vi "setSerializedData.vi"(0 "reference":refnum<class "UseCaseNode.lvclass">, 1 "parent":refnum<class "AbstractNode.lvclass">, 2 "children":refnum<class "AbstractNode.lvclass">[](array[class]), 3 "xmlOut":string, 5 "error in (no error)":errorcluster) -> (14 "reference out":refnum<class "UseCaseNode.lvclass">, 19 "error out":errorcluster)   [LabVIEW 2014, in "UseCaseNode.lvclass"]
doc: "setSerializedData"
uses:
  <resource>/Framework/Providers/Open_GDS/UML/UseCaseNode_class/UseCaseNode.lvclass
  <resource>/Framework/Providers/Open_GDS/UML/AbstractNode_class/AbstractNode.lvclass
  <resource>/Framework/Providers/Open_GDS/UML/General/Rectangle/Rectangle Rectangle2D.ctl
  <resource>/Framework/Providers/Open_GDS/UML/MultiLineString_class/MultiLineString.lvclass
  <resource>/Framework/Providers/Open_GDS/UML/RectangularNode_class/RectangularNode.lvclass
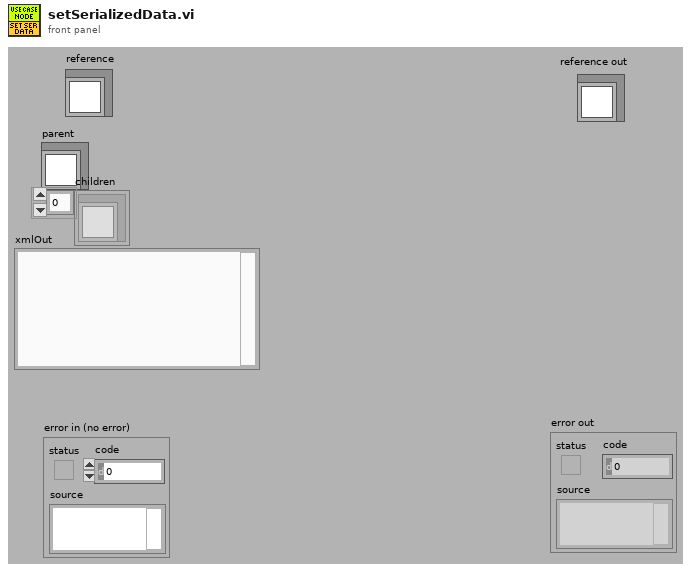
[diagram p1: front panel]
types:
  T1 = typedef "Rectangle Rectangle2D.ctl" = cluster{"x":dbl, "y":dbl, "width":dbl, "height":dbl}
  T2 = cluster{"Base class":cluster{"Base class":cluster{"parent":refnum<k1>, "children":refnum<k1>[]}, "bounds":T1}, "name":refnum<k1>, "DEFAULT_WIDTH":i32, "DEFAULT_HEIGHT":i32}
  T3 = cluster{"Attributes":cluster{"Base class":cluster{"Base class":cluster{"parent":refnum<k1>, "children":refnum<k1>[]}, "bounds":T1}, "name":refnum<k1>, "DEFAULT_WIDTH":i32, "DEFAULT_HEIGHT":i32}, string}
  T4 = typedef "UseCaseNode.lvclass/ObjectAttributes.ctl" = cluster{"name":refnum<class "MultiLineString.lvclass">, "DEFAULT_WIDTH":i32, "DEFAULT_HEIGHT":i32}
  T5 = typedef "RectangularNode.lvclass/ObjectAttributes.ctl" = cluster{"bounds":T1}
  T6 = typedef "AbstractNode.lvclass/ObjectAttributes.ctl" = cluster{"parent":refnum<class "AbstractNode.lvclass">, "children":refnum<class "AbstractNode.lvclass">[], "Hidden":bool}
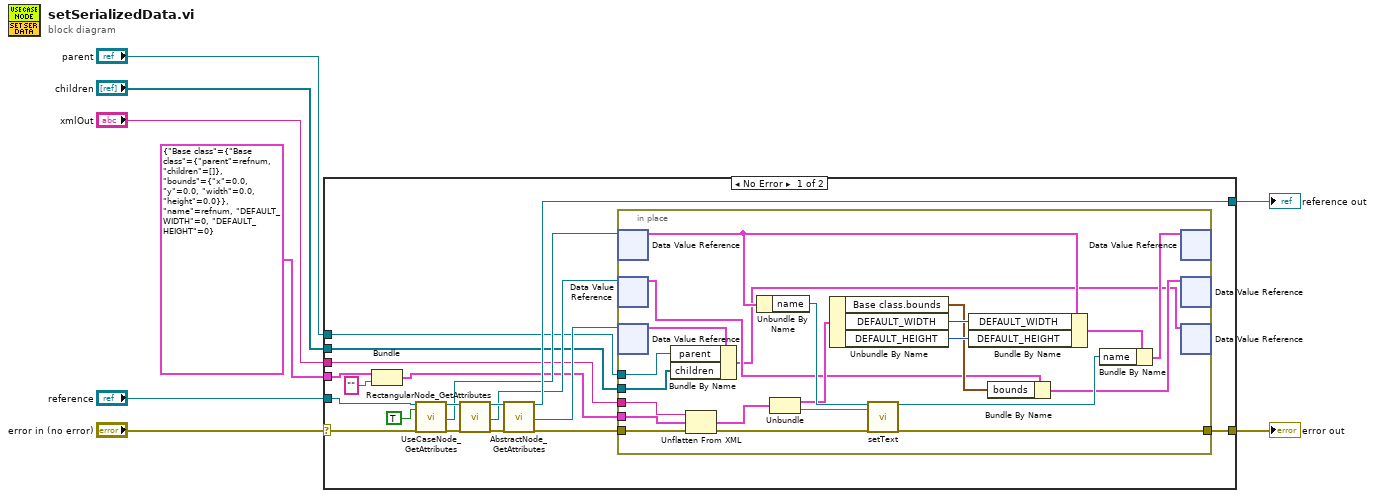
[diagram p0: block diagram]
diagram:
  n1 = case shown="No Error" "error in (no error)" {
    selector: "error in (no error)" -> [w26 w50]
    tunnel: "reference" -> [w27 w51]
    tunnel: [w25 w50] -> w6
    tunnel: [w24 w51] -> w5
    tunnel: "xmlOut" -> [w11 _]
    tunnel: "parent" -> [w10 _]
    tunnel: "children" -> [w9 _]
    tunnel: T2 {"Base class"={"Base class"={"parent"=refnum, "children"=[]}, "bounds"={"x"=0.0, "y"=0.0, "width"=0.0, "height"=0.0}}, "name"=refnum, "DEFAULT_WIDTH"=0, "DEFAULT_HEIGHT"=0} ("Attributes") -> [w22 _]
    frame No Error {
      n2 = Bundle("Attributes"=w22, "") -> (w12:T3)  [unwired: 1 out]
      n3 = call <resource>:"UseCaseNode_GetAttributes.vi"("reference in"=w27, "OnlyGetDvrReference(False)"=TRUE, "error in (no error)"=w26) -> ("reference out"=w20:refnum<class "UseCaseNode.lvclass">, "DataRef"=w16:refnum<data-value>, "error out"=w19:errorcluster)  [unwired: 13 in, 1 out]
      n4 = call <resource>:"RectangularNode_GetAttributes.vi"("reference in"=w20, "error in (no error)"=w19) -> ("reference out"=w18:refnum<class "UseCaseNode.lvclass">, "DataRef"=w15:refnum<data-value>, "error out"=w17:errorcluster)  [unwired: 14 in, 1 out]
      n5 = call <resource>:"AbstractNode_GetAttributes.vi"("reference in"=w18, "error in (no error)"=w17) -> ("reference out"=w24:refnum<class "UseCaseNode.lvclass">, "DataRef"=w14:refnum<data-value>, "error out"=w13:errorcluster)  [unwired: 14 in, 1 out]
      n6 = in-place {
        in-place-border: [w38] -> w25
        in-place-border: w13 -> [w35]
        in-place-border: w12 -> [w34]
        in-place-border: w11 -> [w33]
        in-place-border: w10 -> [w30]
        in-place-border: w9 -> [w29]
        n7 = in-place-dvr #1(w16) -> (w49:T4)  [unwired: 1 out]
        n8 = in-place-dvr #2(w15) -> (w36:T5)  [unwired: 1 out]
        n9 = in-place-dvr #3(w14) -> (w31:T6)  [unwired: 1 out]
        n10 = Bundle By Name(cluster=w31, "parent"=w30, "children"=w29) -> (w28:T6)
        n11 = Unflatten From XML(xml string=w33, type=w34, error in (no error)=w35) -> (value=w37:T3, error out=w39:errorcluster)
        n12 = Unbundle By Name(w49) -> ("name"=w45:refnum<class "MultiLineString.lvclass">)
        n13 = Unbundle(w37) -> ("Attributes"=w42:T2, w40:string)
        n14 = Unbundle By Name(w42) -> ("Base class.bounds"=w41:T1, "DEFAULT_WIDTH"=w48:i32, "DEFAULT_HEIGHT"=w47:i32)
        n15 = call-dynamic "setText.vi"("reference"=w45, "text"=w40, "error in (no error)"=w39) -> ("reference out"=w44:refnum<class "MultiLineString.lvclass">, "error out"=w38:errorcluster)  [unwired: 15 out]
        n16 = Bundle By Name(cluster=w49, "DEFAULT_WIDTH"=w48, "DEFAULT_HEIGHT"=w47) -> (w46:T4)
        n17 = Bundle By Name(cluster=w36, "bounds"=w41) -> (w32:T5)
        n18 = Bundle By Name(cluster=w46, "name"=w44) -> (w43:T4)
        n19 = in-place-dvr #1(w43) -> ()  [unwired: 2 out]
        n20 = in-place-dvr #2(w32) -> ()  [unwired: 2 out]
        n21 = in-place-dvr #3(w28) -> ()  [unwired: 2 out]
      }
    }
    frame Error {
    }
  }
  "reference out" <- w5
  "error out" <- w6
